vi "Idle_Action.vi"(5 "GuiRef":T1, 8 "error in":errorcluster, 9 "IdentifyReady":refnum<vi>) -> (0 "error out":errorcluster, 3 "SlotReady":bool)   [LabVIEW 2013]
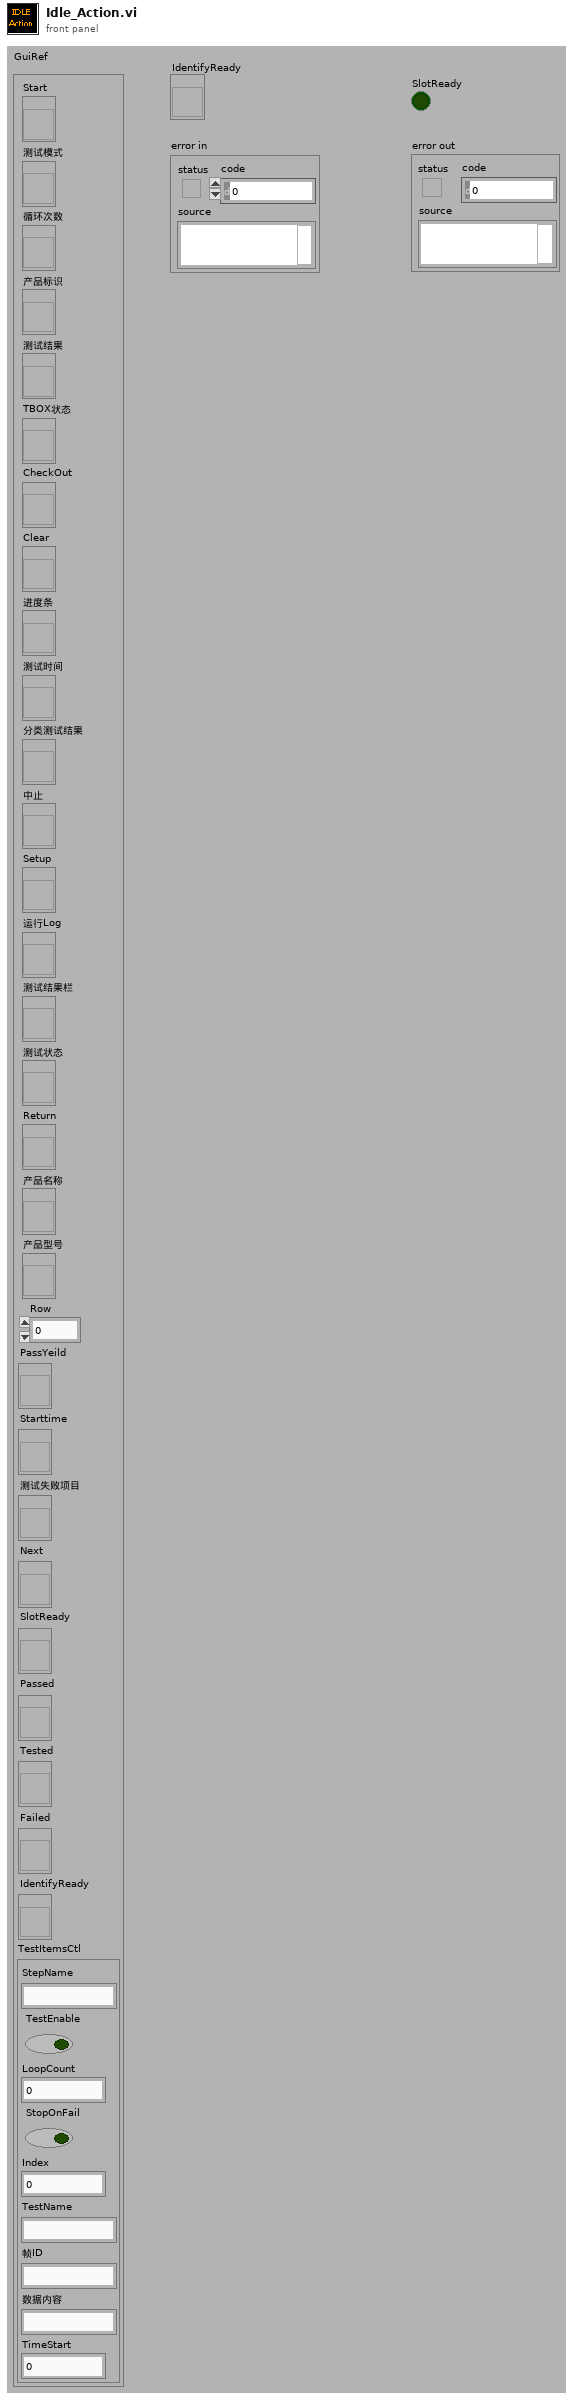
[diagram p1: front panel]
types:
  T1 = typedef "控件.ctl" = cluster{"Start":refnum<vi>, "测试模式":refnum<vi>, "循环次数":refnum<vi>, "产品标识":refnum<vi>, "测试结果":refnum<vi>, "TBOX状态":refnum<vi>, "CheckOut":refnum<vi>, "Clear":refnum<vi>, "进度条":refnum<vi>, "测试时间":refnum<vi>, "分类测试结果":refnum<vi>, "中止":refnum<vi>, "Setup":refnum<vi>, "运行Log":refnum<vi>, "测试结果栏":refnum<vi>, "测试状态":refnum<vi>, "Return":refnum<vi>, "产品名称":refnum<vi>, "产品型号":refnum<vi>, "Row":i32, "PassYeild":refnum<vi>, "Starttime":refnum<vi>, "测试失败项目":refnum<vi>, "Next":refnum<vi>, "SlotReady":refnum<vi>, "Passed":refnum<vi>, "Tested":refnum<vi>, "Failed":refnum<vi>, "IdentifyReady":refnum<vi>, "TestItemsCtl":cluster{"StepName":string, "TestEnable":bool, "LoopCount":u32, "StopOnFail":bool, "Index":u32, "TestName":string, "帧ID":string, "数据内容":string, "TimeStart":u32}}
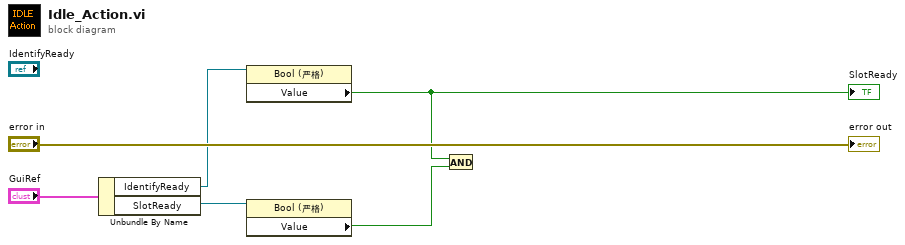
[diagram p0: block diagram]
diagram:
  n1 = Unbundle By Name("GuiRef") -> ("IdentifyReady"=w1:refnum<vi>, "SlotReady"=w3:refnum<vi>)
  n2 = property class="Bool (严格)"(reference=w1) -> ("Value"=w5:bool)  [unwired: 1 in, 2 out]
  "SlotReady" <- w5
  n3 = property class="Bool (严格)"(reference=w3) -> ("Value"=w2:bool)  [unwired: 1 in, 2 out]
  n4 = And(x=w5, y=w2) -> ()  [unwired: 1 out]
  "error out" <- "error in"
